vi "avaerage_attempt.vi"() -> ()   [LabVIEW 2020]
panel:
  out "Waveform Chart":dbl(graph)
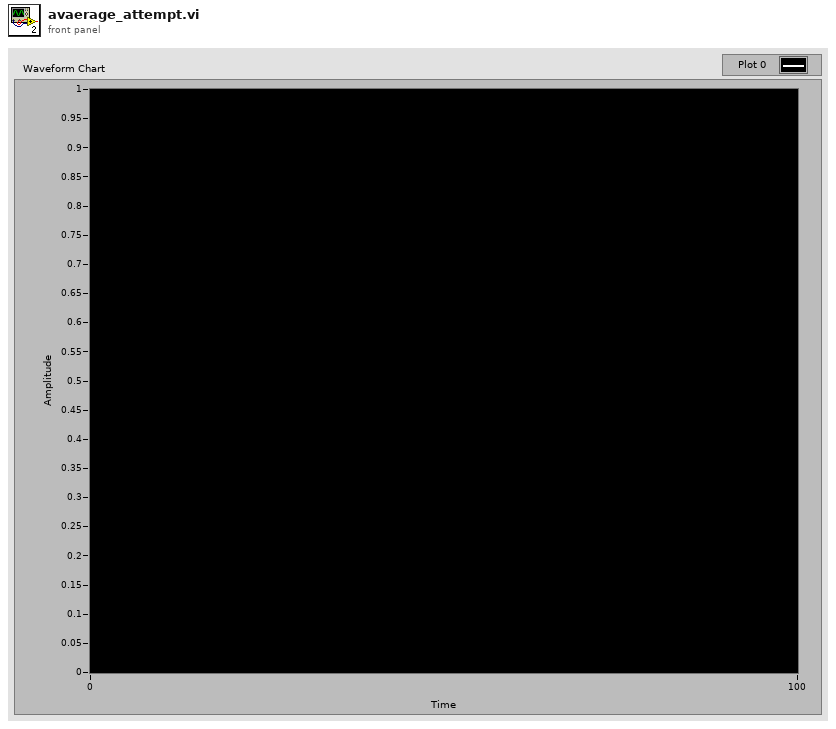
[diagram p1: front panel]
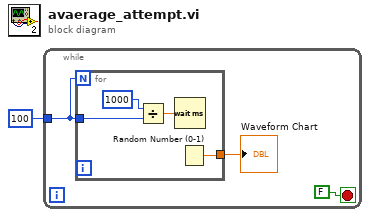
[diagram p0: block diagram]
diagram:
  n1 = while {
    tunnel: 100 -> [w2]
    stop <- FALSE stop-if-true
    n2 = for {
      N: w2 -> [_]
      tunnel: [w8] -> w4
      tunnel: w2 -> [w5]
      n3 = Divide(x=u32 1000 ("milliseconds to wait"), y=w5) -> (x/y=w6:dbl)
      n4 = Wait (ms)(milliseconds to wait=w6) -> ()  [unwired: 1 out]
      n5 = Random Number (0-1)() -> (number: 0 to 1=w8:dbl)
    }
    "Waveform Chart" <- w4
  }
